vi "Gray if False.vi"(1 "Checkbox":bool) -> (0 "Enabled":T1(ring))   [LabVIEW 2015, in "Endigit.lvlib"]
doc: "Returns the enum value \"Disabled and Grayed Out\" if \"Checkbox\" is false.\n\nAuthored by Robert C. Mortensen\nrobert@endigit.com\n\nCopyright (c) 2015, Endigit, Inc."
uses:
  Endigit.lvlib
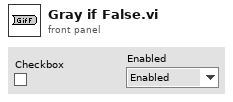
[diagram p1: front panel]
types:
  T1 = enum8{"Enabled", "Disabled", "Disabled and Grayed Out"}
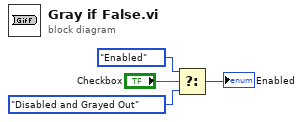
[diagram p0: block diagram]
diagram:
  n1 = Select(t=T1."Enabled" ("Disabled"), s="Checkbox", f=T1."Disabled and Grayed Out" ("Disabled")) -> (s? t:f=→"Enabled":T1)
